vi "二极管的伏安特性曲线.vi"() -> ()   [LabVIEW 2017]
panel:
  out "XY Graph":cluster{"X":dbl[], "Y":dbl[]}[](graph)
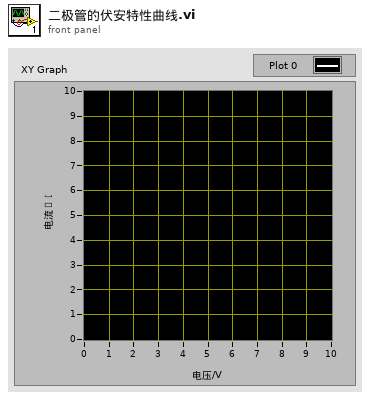
[diagram p1: front panel]
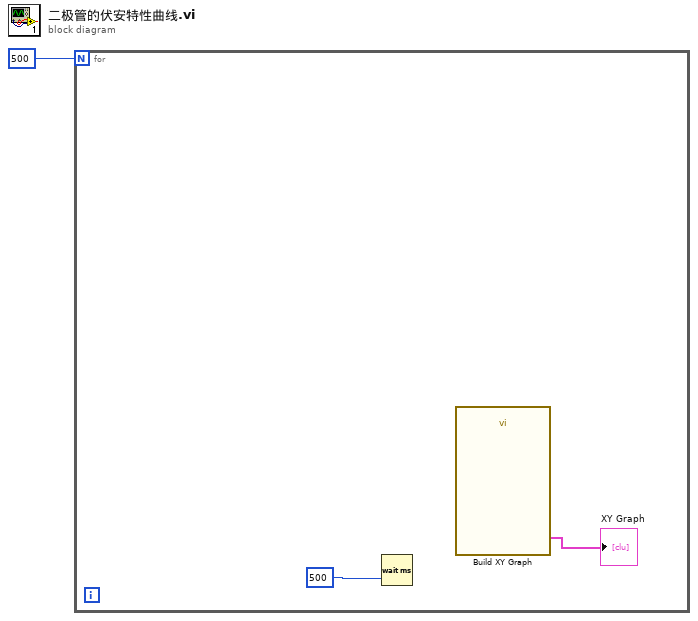
[diagram p0: block diagram]
diagram:
  n1 = for {
    N: 500 -> [_]
    n2 = Wait (ms)(milliseconds to wait=500) -> ()  [unwired: 1 out]
    n3 = call "Build XY Graph"() -> ("XY Graph"=→"XY Graph":cluster{"X":dbl[], "Y":dbl[]}[])  [unwired: 10 in, 1 out]
  }
